vi "setICImagingControlRef.vi"(8 "error in (no error)":errorcluster, 10 "ICImagingControlRef":refnum<k7>, 11 "ICCameraAcquisitor.lvclass in":refnum<class "ICCameraAcquisitor.lvclass">) -> (0 "error out":errorcluster, 3 "ICCameraAcquisitor.lvclass out":refnum<class "ICCameraAcquisitor.lvclass">)   [LabVIEW 2011, in "Hardware.lvlib" / "Channels.lvlib" / "ICCameraAcquisitor.lvclass"]
uses:
  ICCameraAcquisitor.lvclass
  ICCameraAcquisitor.lvclass/ICCameraAcquisitor.ctl
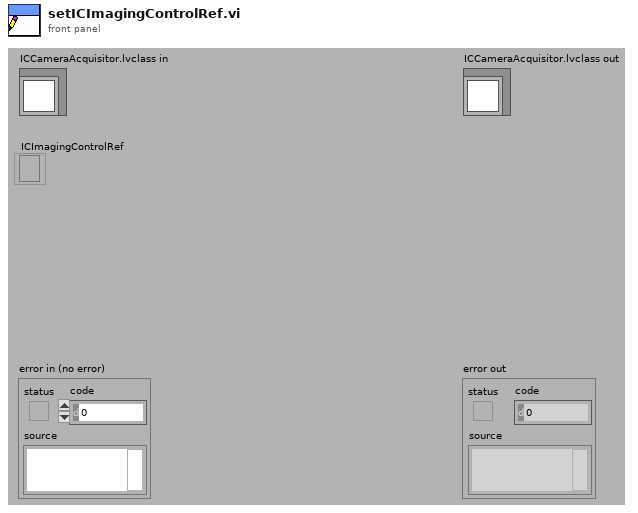
[diagram p1: front panel]
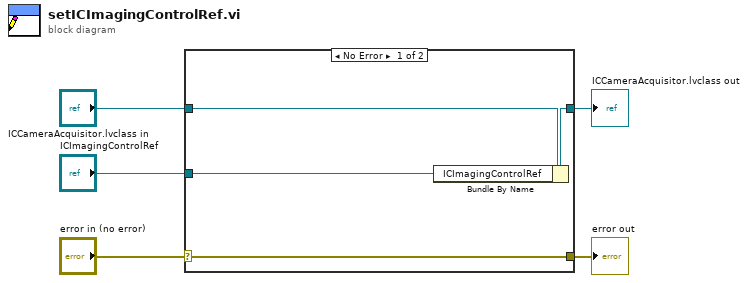
[diagram p0: block diagram]
diagram:
  n1 = case shown="No Error" "error in (no error)" {
    selector: "error in (no error)" -> [w9 w10]
    tunnel: [w9 w10] -> w4
    tunnel: [w7 w11] -> w2
    tunnel: "ICCameraAcquisitor.lvclass in" -> [w8 w11]
    tunnel: "ICImagingControlRef" -> [w6 _]
    frame No Error {
      n2 = Bundle By Name(cluster=w8, "ICImagingControlRef"=w6) -> (w7:refnum<class "ICCameraAcquisitor.lvclass">)
    }
    frame Error {
    }
  }
  "error out" <- w4
  "ICCameraAcquisitor.lvclass out" <- w2
